vi "AttrGetTxTotal.vi"(8 "error in":errorcluster, 11 "CanHandleIn":T1) -> (0 "error out":errorcluster, 2 "Value":u32, 3 "CanHandleOut":T1)   [LabVIEW 2011, in "Konvolucio MCAN120803.lvlib"]
uses:
  <instrlib>/Konvolucio MCAN120803/Konvolucio MCAN120803.lvlib
  <instrlib>/Konvolucio MCAN120803/Types/CanHandleType.ctl
  C:/Program Files/National Instruments/LabVIEW 2011/instr.lib/Konvolucio MCAN120803/Private/Konvolucio.MCAN120803.API.dll
  Private/Konvolucio.MCAN120803.API.dll
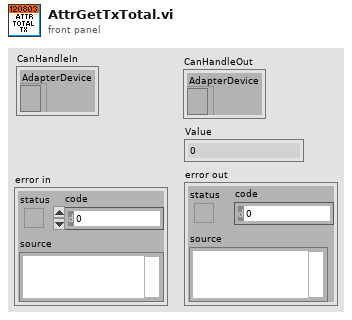
[diagram p1: front panel]
types:
  T1 = typedef "Konvolucio MCAN120803.lvlib/CanHandleType.ctl" = cluster{"AdapterDevice":refnum<k24>}
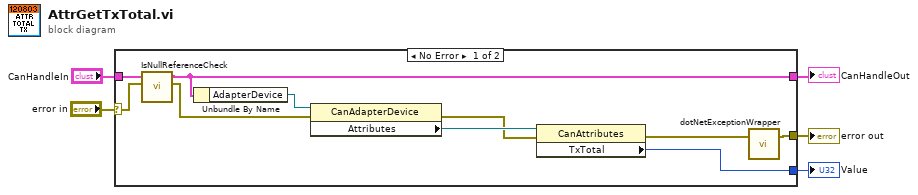
[diagram p0: block diagram]
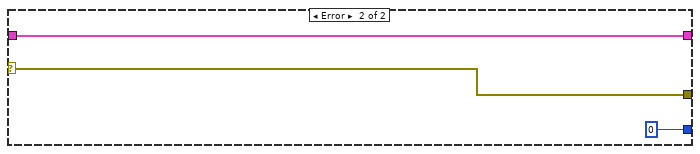
[diagram p2: hidden frame]
diagram:
  n1 = case shown="No Error" "error in" {
    selector: "error in" -> [w11 w18]
    tunnel: [w14 w18] -> w5
    tunnel: [w15 u32 0 ("Attributes.RxErrorCounter")] -> w3
    tunnel: [w10 w16] -> w2
    tunnel: "CanHandleIn" -> [w12 w16]
    frame No Error {
      n2 = call <instrlib>:"IsNullReferenceCheck.vi"("error in"=w11, "MCanHandleIn"=w12) -> ("error out"=w8:errorcluster, "MCanHandleOut"=w10:T1)  [unwired: 5 in]
      n3 = Unbundle By Name(w10) -> ("AdapterDevice"=w9:refnum<k24>)
      n4 = property class="CanAdapterDevice"(reference=w9, error in=w8) -> (error out=w6:errorcluster, "Attributes"=w7:refnum<k24>)  [unwired: 1 out]
      n5 = property class="CanAttributes"(reference=w7, error in=w6) -> (error out=w13:errorcluster, "TxTotal"=w15:u32)  [unwired: 1 out]
      n6 = call <instrlib>:"dotNetExceptionWrapper.vi"("error in"=w13) -> ("error out"=w14:errorcluster)  [unwired: 2 in]
    }
    frame Error {
    }
  }
  "error out" <- w5
  "Value" <- w3
  "CanHandleOut" <- w2
